vi "DMMP_GetSamplingRate.vi"(3 "Input DMMP":refnum<class "DMMP.lvclass">) -> (0 "Sampling Rate (point / sec)":u32, 1 "Output DMMP":refnum<class "DMMP.lvclass">)   [LabVIEW 2014, in "DMMP.lvclass"]
uses:
  DMMP.lvclass
  DMMP.lvclass/DMMP.ctl
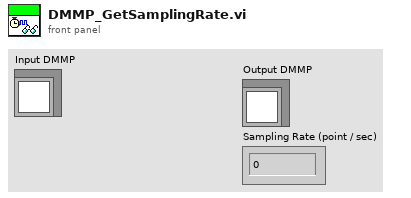
[diagram p1: front panel]
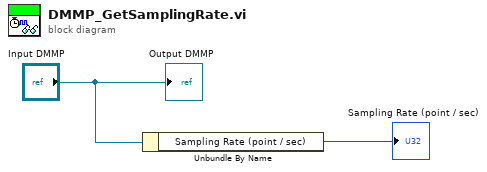
[diagram p0: block diagram]
diagram:
  n1 = Unbundle By Name("Input DMMP") -> ("Sampling Rate (point / sec)"=→"Sampling Rate (point / sec)":u32)
  "Output DMMP" <- "Input DMMP"
